vi "03-QNET_MECHKIT_Piezo.vi"() -> ()   [LabVIEW 2012]
doc: "This VI is to be used with the NI-ELVIS and the QNET-Mechatronic Sensors I module. The objective is to learn about how the Piezo sensor works and find the natural frequency of the attached weight."
uses:
  <vilib>/Simulation/Scripting/Companion Diagram/SimConfigNode/SimParams.ctl
  <vilib>/Simulation/Scripting/Companion Diagram/SimConfigNode/_simSolvers.ctl
  <vilib>/Simulation/Implementation/Shared/SIMSCR Execution Mode.ctl
  <vilib>/Simulation/Param Hierarchy/Typedefs/SIMPH Param Control Actions.ctl
  <vilib>/Simulation/Implementation/Shared/NILVSim_ParamChanged.vi
  <vilib>/Simulation/Utility/Implementation/NILVSim Collector.llb/SIM Collector (scalar).vi
  <vilib>/Simulation/SignalDisplay/Implementation/NILVSim Time Waveform.llb/SIM Time Waveform (scalar).vi
  <vilib>/Simulation/Utility/Implementation/SIM Halt.vi
  <vilib>/Simulation/Implementation/Shared/NILVSim_Manager.vi
  <vilib>/Simulation/Implementation/Shared/NILVSim_FinalizeModel.vi
  <vilib>/Simulation/Utility/Implementation/NILVSim Collector.llb/NILVSim Collector core (scalar).vi
  <vilib>/Simulation/Implementation/Shared/SIM Unbundle Sim Info.vi
  <vilib>/Utility/error.llb/Clear Errors.vi
  <vilib>/Simulation/Implementation/Shared/NILVSim_GetModelError.vi
  <vilib>/Simulation/Implementation/Shared/SIM Bundle Sim Info.vi
  <vilib>/Simulation/Implementation/Shared/SIMSH Read Queue.vi
  <vilib>/Simulation/Implementation/Shared/NILVSim_Initialize.vi
  <vilib>/DAQmx/read.llb/DAQmx Read.vi
  <vilib>/DAQmx/read.llb/DAQmx Read (Analog DBL 1Chan 1Samp).vi
  <vilib>/Simulation/Utility/Implementation/NILVSim Get Time and IsAcceptedStep.vi
  <vilib>/express/express analysis/Spectral/Block/exnSpectralBlock spectral measurements power poly.vi
  <vilib>/express/express analysis/Spectral/Block/exnSpectralBlock spectral measurements power WFM.vi
  <vilib>/Simulation/Scripting/Companion Diagram/SimConfigNode/SimDog.xnode
  <vilib>/Simulation/Implementation/XNodeFramework/SimXNode/SimX.xnode
  <vilib>/express/express analysis/Spectral/XNode/ExpressSpectralMeasurementsBlockNode.xnode
  <vilib>/Simulation/Implementation/Shared/NI_SIM_Implementation.lvlib
panel:
  in  "Sampling Rate (Hz)":dbl=100.0 min=0.0 max=1000.0 step=25.0 format="%.1f"
  in  "Device":tag="Dev1"
  in  "Tab Control":enum32{"Collect Data", "Natural Frequency"}(tab)
  out "Piezo (V)":waveform(dbl)(graph)
  out "Power Spectrum":cluster{"f0":dbl, "df":dbl, "magnitude":dbl[]}(graph)
  in  "stop":bool
  # "QNET-MECHKIT Piezo"
  # "NOTE: Place J8 jumper on \"Piezo\" setting."
  # "Perturb the Piezo sensor and examine the obtained response."
  # "1) Perturb the Piezo manually.\n2) Once it stopped resonating, click on the STOP button to stop running the VI.\n3) The spectrum is shown below."
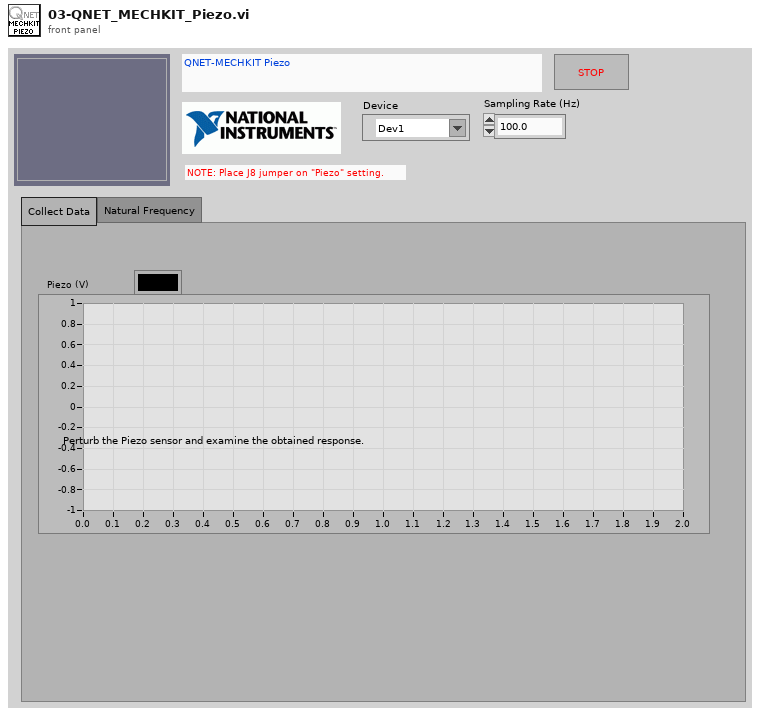
[diagram p1: front panel]
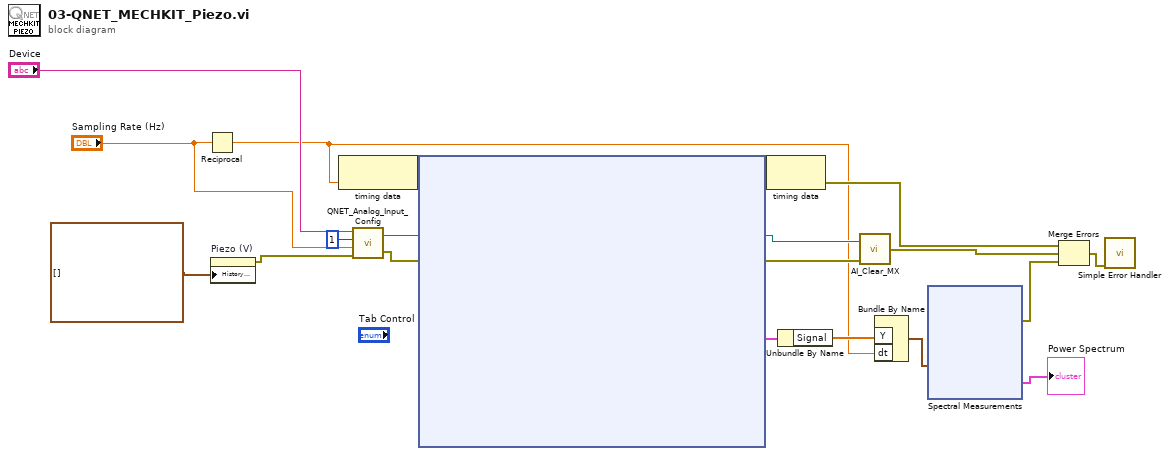
[diagram p0: block diagram]
diagram:
  n1 = Reciprocal(x="Sampling Rate (Hz)") -> (1/x=w4:dbl)
  n2 = property on="Piezo (V)" class="WFChart (strict)"("History Data"=waveform(dbl)[] []) -> (error out=w6:errorcluster)  [unwired: 2 in, 1 out]
  n3 = node-c288(w4) -> (w19:variant)
  n4 = call "QNET_Analog_Input_Config.vi"("error in"=w6, "sampling rate (Hz)"="Sampling Rate (Hz)", "analog input channel"=u32 1, "dev"="Device") -> ("error out"=w16:errorcluster, "task out"=w15:refnum<k21>)
  n5 = node-c254 ("Simulation Loop")(w19, w16, w15) -> (w18:variant, w14:refnum<k21>, w13:errorcluster, w11:cluster{"Time":dbl[], "Signal":dbl[]})
  n6 = node-c288(w18) -> (w10:errorcluster)
  n7 = Unbundle By Name(w11) -> ("Signal"=w5:dbl[])
  n8 = call "AI_Clear_MX.vi"("Error in"=w13, "Task in"=w14) -> ("Error out"=w9:errorcluster)
  n9 = Bundle By Name("Y"=w5, "dt"=w4) -> (w3:waveform(dbl))  [unwired: 1 out]
  n10 = xnode "Spectral Measurements"("Signals"=w3) -> ("Power Spectrum"=→"Power Spectrum":cluster{"f0":dbl, "df":dbl, "magnitude":dbl[]}, "error out"=w1:errorcluster)  [unwired: 1 in]
  n11 = Merge Errors(w10, w9, w1) -> (w8:errorcluster)
  n12 = call <vilib>:"Simple Error Handler.vi"("error in (no error)"=w8) -> ()  [unwired: 1 in, 8 out]
